vi "Expt9 niUSRP EX PSK Tx.vi"() -> ()   [LabVIEW 2020]
doc: "This example <B>requires the Modulation Toolkit</B>.\n\nApplies PSK (Phase Shift Keyed Modulation) to a PN sequence for USRP-based transmission. Continuously transmits a repeating message with a length determined by the PN Sequence Order parameter. \n\nThis example is paired with the example \"niUSRP Ex PSK Rx.vi\", which allows you to establish a Tx / Rx link between two separate USRPs. \n\nTo establish a Tx / Rx link between two USRPs:\n1) Ensure that the Tx and Rx example VIs have matching parameters for Modulation Scheme (M-Ary), Carrier Frequency, and Symbol Rate. Specify the Symbol Rate by setting the combination of the IQ Sampling Rate and the Number of Samples per Symbol parameters.\n2) Choose an IQ Sample Rate that enables sufficient Rx bandwidth.\n3) Set the Tx and / or Rx gain to ensure a sufficient signal to noise ratio on the Receive side. Note: applying too much gain can result in clipping.\n4) Choose a sufficient acquisition frame length to enable the demodulator to lock to the transmitted signal. National Instruments recommends that the acquired frame contain a number of symbols that is at least 20 * M-Ary of the modulation scheme. \n5) Ensure that the Reset Demodulator control is set to True until a solid lock is established. \n6) Install antennas and attenuators that efficiently operate at the carrier frequency you choose."
uses:
  <vilib>/addons/Modulation/Digital/General/MT Generate PSK System Parameters(M).vi
  <instrlib>/niUSRP/niUSRP Write Tx Data (CDB Cluster).vi
  <vilib>/addons/Modulation/niDMT.lvlib
panel:
  out "error out":errorcluster
  in  "Enabled Channel":string(combo)="0"
  out "Gain [dB] (actual)":dbl=12.0 format="%#.6p"
  out "Carrier Frequency \n[Hz] (actual)":dbl=915000000.0 format="%#.6p"
  out "IQ Sampling\nRate [S/sec] (actual)":dbl=500000.0 format="%#.6p"
  in  "Active Antenna":string(combo)="TX1"
  in  "Gain [dB]":dbl=12.0 format="%#.6p"
  in  "Carrier\nFrequency [Hz]":dbl=915000000.0 format="%#.6p"
  in  "IQ Sampling\nRate [S/sec]":dbl=500000.0 format="%#.6p"
  in  "Device Name":refnum<k15>="192.168.10.5"
  in  "Choose a PSK Format":T1(tab)=enum."8-PSK" caption="PSK"
  in  "BPSK System Parameters":T2={"Samples per Symbol"=8, "symbol map"=[], "Differential PSK"=enum."disable", "PSK type"=0} {"PSK type" items=["normal", "shifted", "offset"]; "symbol map" format="%.3f"}
  in  "QPSK System Parameters":T2={"Samples per Symbol"=8, "symbol map"=[], "Differential PSK"=enum."disable", "PSK type"=0} {"PSK type" items=["normal", "shifted", "offset"]; "symbol map" format="%.3f"}
  in  "pi/4 DQPSK System Parameters":T2={"Samples per Symbol"=8, "symbol map"=[], "Differential PSK"=enum."enable", "PSK type"=1} {"PSK type" items=["normal", "shifted", "offset"]; "symbol map" format="%.3f"}
  in  "OQPSK System Parameters":T2={"Samples per Symbol"=8, "symbol map"=[], "Differential PSK"=enum."disable", "PSK type"=2} {"PSK type" items=["normal", "shifted", "offset"]; "symbol map" format="%.3f"}
  in  "8-PSK System Parameters":T2={"Samples per Symbol"=4, "symbol map"=[], "Differential PSK"=enum."disable", "PSK type"=0} {"PSK type" items=["normal", "shifted", "offset"]; "symbol map" format="%.3f"}
  in  "16-PSK System Parameters":T2={"Samples per Symbol"=8, "symbol map"=[], "Differential PSK"=enum."disable", "PSK type"=0} {"PSK type" items=["normal", "shifted", "offset"]; "symbol map" format="%.3f"}
  in  "M":i32=4 min=2 step=2
  in  "Custom System Parameters":T2={"Samples per Symbol"=8, "symbol map"=[], "Differential PSK"=enum."disable", "PSK type"=0} {"PSK type" items=["normal", "shifted", "offset"]; "symbol map" format="%.3f"}
  out "Frame Size [samples]":i32=4092
  in  "Pn Sequence Order":i32=13
  in  "Filter Parameters":T3={"Alpha"=0.5, "Filter Length"=6, "TX Filter"=enum."Root Raised Cos"} {"Alpha" format="%.2f"}
  out "Symbol Rate\n[symbols/sec]":dbl=500000.0 format="%#.6p"
  in  "Stop":bool
  out "Constellation Graph":T4(graph) caption="Tx Signal Constellation"
  # "Note:\nFrame size (samples per write) =\n (2^Pn Sequence Order) * Samples Per Symbol.\nUse Pn Sequence Order of 12 when using a 1 Gb Ethernet connection on a USRP RIO device. This prevents underflows by implicitly choosing \na frame size close to the ideal frame size for Ethernet connection. Refer to the \"Data Streaming Performance Tips\" section in the NI-USRP Help at ni.com/manuals for more information."
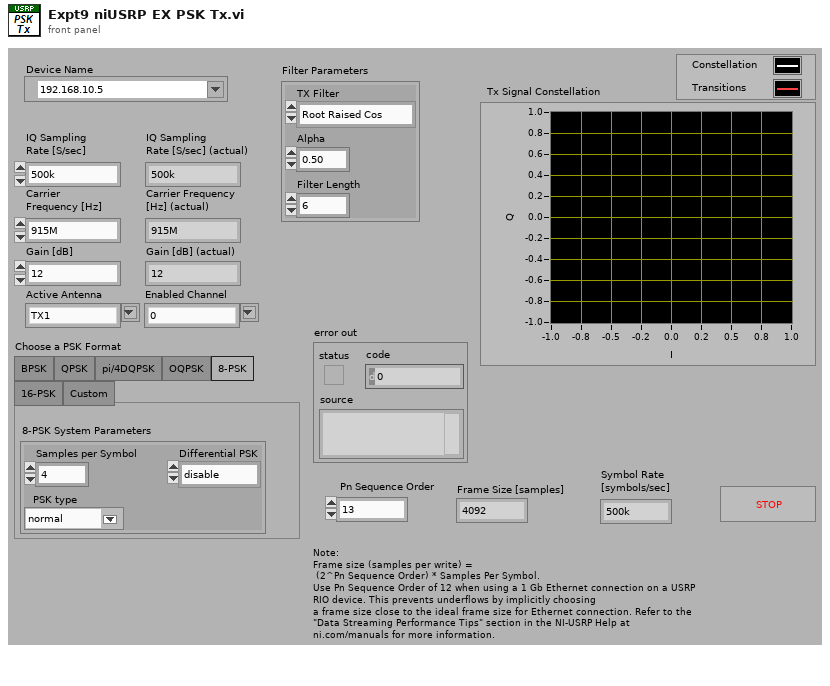
[diagram p1: front panel]
types:
  T1 = enum32{"BPSK", "QPSK", "pi/4DQPSK", "OQPSK", "8-PSK", "16-PSK", "Custom"}
  T2 = cluster{"Samples per Symbol":i32, "symbol map":cdb[], "Differential PSK":enum16{"disable", "enable"}, "PSK type":u16}
  T3 = cluster{"Alpha":dbl, "Filter Length":i32, "TX Filter":enum16{"none", "Raised Cosine", "Root Raised Cos", "Gaussian"}}
  T4 = cluster{"constellation":dbl[], "oversampled data":dbl[]}[]
  T5 = enum32{"PN sequence", "user-defined pattern", "Read from file"}
  T6 = cluster{"samples per symbol (16)":i32, "symbol map":cdb[], "differential PSK":enum16{"disable", "enable"}, "PSK type":u16}
  T7 = typedef "niAMT.lvlib/Complex Data Waveform.ctl" = cluster{"t0":dbl, "dt":dbl, "Y":cdb[]}
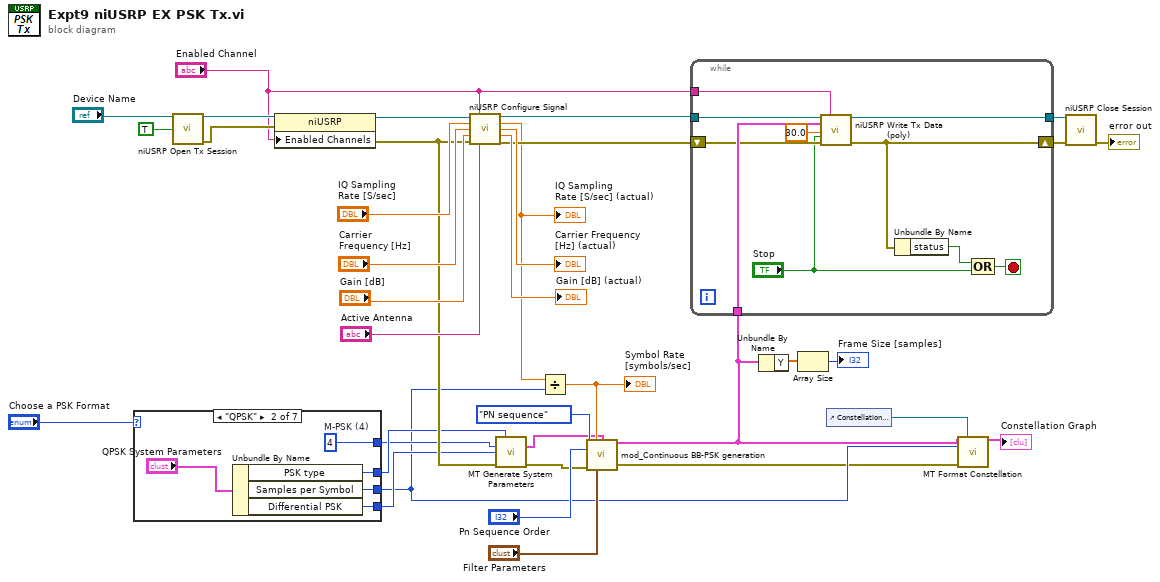
[diagram p0: block diagram]
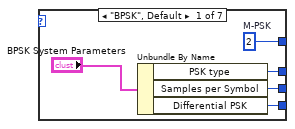
[diagram p2: hidden frame]
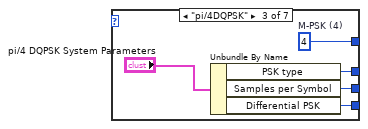
[diagram p3: hidden frame]
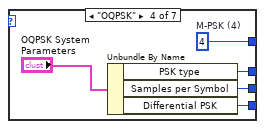
[diagram p4: hidden frame]
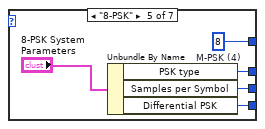
[diagram p5: hidden frame]
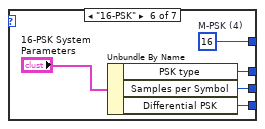
[diagram p6: hidden frame]
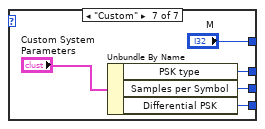
[diagram p7: hidden frame]
diagram:
  n1 = case shown="\"QPSK\"" "Choose a PSK Format" {
    tunnel: [w38 w45 w50 w55 w60 w66 w69] -> w4
    tunnel: [w39 w43 w49 w54 w59 w65 w70] -> w7
    tunnel: [w41 w46 w51 w56 w58 w64 "M"] -> w6
    tunnel: [w40 w44 w48 w53 w61 w63 w71] -> w8
    frame "BPSK", Default {
      w41 = 2  # M-PSK
      n2 = Unbundle By Name("BPSK System Parameters") -> ("PSK type"=w40:u16, "Samples per Symbol"=w38:i32, "Differential PSK"=w39:enum16{"disable", "enable"})
    }
    frame "QPSK" {
      w46 = 4  # M-PSK (4)
      n3 = Unbundle By Name("QPSK System Parameters") -> ("PSK type"=w44:u16, "Samples per Symbol"=w45:i32, "Differential PSK"=w43:enum16{"disable", "enable"})
    }
    frame "pi/4DQPSK" {
      w51 = 4  # M-PSK (4)
      n4 = Unbundle By Name("pi/4 DQPSK System Parameters") -> ("PSK type"=w48:u16, "Samples per Symbol"=w50:i32, "Differential PSK"=w49:enum16{"disable", "enable"})
    }
    frame "OQPSK" {
      w56 = 4  # M-PSK (4)
      n5 = Unbundle By Name("OQPSK System Parameters") -> ("PSK type"=w53:u16, "Samples per Symbol"=w55:i32, "Differential PSK"=w54:enum16{"disable", "enable"})
    }
    frame "8-PSK" {
      w58 = 8  # M-PSK (4)
      n6 = Unbundle By Name("8-PSK System Parameters") -> ("PSK type"=w61:u16, "Samples per Symbol"=w60:i32, "Differential PSK"=w59:enum16{"disable", "enable"})
    }
    frame "16-PSK" {
      w64 = 16  # M-PSK (4)
      n7 = Unbundle By Name("16-PSK System Parameters") -> ("PSK type"=w63:u16, "Samples per Symbol"=w66:i32, "Differential PSK"=w65:enum16{"disable", "enable"})
    }
    frame "Custom" {
      n8 = Unbundle By Name("Custom System Parameters") -> ("PSK type"=w71:u16, "Samples per Symbol"=w69:i32, "Differential PSK"=w70:enum16{"disable", "enable"})
    }
  }
  n9 = call <instrlib>:"niUSRP Open Tx Session.vi"("device names"="Device Name", "reset"=TRUE) -> ("session handle out"=w16:refnum<k15>, "error out"=w15:errorcluster)  [unwired: 12 in]
  n10 = property class="niUSRP"(reference=w16, error in=w15, "Enabled Channels"="Enabled Channel") -> (reference out=w14:refnum<k15>, error out=w10:errorcluster)
  n11 = call <instrlib>:"niUSRP Configure Signal.vi"("session handle"=w14, "channel list"="Enabled Channel", "IQ rate"="IQ Sampling\nRate [S/sec]", "carrier frequency"="Carrier\nFrequency [Hz]", "gain"="Gain [dB]", "error in (no error)"=w10, "active antenna"="Active Antenna") -> ("session handle out"=w19:refnum<k15>, "coerced IQ rate"=w17:dbl, "coerced carrier frequency"=→"Carrier Frequency \n[Hz] (actual)":dbl, "coerced gain"=→"Gain [dB] (actual)":dbl, "error out"=w18:errorcluster)  [unwired: 4 in]
  "IQ Sampling\nRate [S/sec] (actual)" <- w17
  n12 = call-poly <vilib>:"MT Generate System Parameters.vi"("PSK type"=w8, "M-PSK (4)"=w6, "differential PSK"=w7, "error in (no error)"=w10) -> ("PSK system parameters"=w9:T6, "error out"=w11:errorcluster)  [unwired: 9 in, 1 out]
  n13 = Divide(x=w17, y=w4) -> (x/y=w30:dbl)
  "Symbol Rate\n[symbols/sec]" <- w30
  n14 = call <vilib>:"mod_Continuous BB-PSK generation.vi"("bit stream type"=T5."PN sequence", "Symbol Rate, Hz"=w30, "Custom-PSK Parameters"=w9, "PN Sequence Order"="Pn Sequence Order", "error in (no error)"=w11, "filter parameters"="Filter Parameters") -> ("output complex waveform"=w5:T7, "error out"=w3:errorcluster)  [unwired: 7 in, 1 out]
  n15 = while {
    tunnel: [w78] -> w28
    tunnel: w19 -> [w81]
    shift-right: [w74] -> w29
    shift-left: w18 -> [w79]
    tunnel: w5 -> [w80]
    tunnel: "Enabled Channel" -> [w73]
    stop <- w77 stop-if-true
    n16 = call-poly <instrlib>:"niUSRP Write Tx Data (poly).vi"("session handle"=w81, "channel list"=w73, "data"=w80, "timeout"=30.0, "end of data?"="Stop", "error in (no error)"=w79) -> ("session handle out"=w78:refnum<k15>, "error out"=w74:errorcluster)  [unwired: 8 in]
    n17 = Unbundle By Name(w74) -> ("status"=w76:bool)
    n18 = Compound Arithmetic op=OR(w76, "Stop") -> (w77:bool)
  }
  n19 = Unbundle By Name(w5) -> ("Y"=w36:cdb[])
  n20 = Array Size(array=w36) -> (size(s)=→"Frame Size [samples]":i32)
  n21 = control-ref of="Constellation Graph"() -> (w1:refnum<vi>)
  n22 = call <vilib>:"MT Format Constellation.vi"("waveform"=w5, "constellation reference"=w1, "samples per symbol"=w4, "error in (no error)"=w3) -> ("constellation graph"=→"Constellation Graph":T4)  [unwired: 10 in, 1 out]
  n23 = call <instrlib>:"niUSRP Close Session.vi"("session handle"=w28, "error in (no error)"=w29) -> ("error out"=→"error out":errorcluster)  [unwired: 13 in]
